vi "MM6.set Special.vi"(0 "i ref in":refnum<vi>, 1 "ms timeout (10000)":i32=10000, 2 "Object":string, 3 "Special":string, 5 "error in (no error)":errorcluster) -> (14 "i ref out":refnum<vi>, 18 "timed out":bool, 19 "error out":errorcluster)   [LabVIEW 2014, in "MM6.lvlib"]
doc: "This VI calls the function \"SetSpecial\" of the object with a certain \"name\" if the Special parameter is not empty nor starting with an asterisk."
uses:
  MM6.lvlib
  CS_Core/CSSystem/CoreDefs/CoreDefs.error_type.ctl
  CS_Core/CSSystem/CoreDefs/CoreDefs.error_severity.ctl
  CS_Core/CSSystem/CoreLib/CoreLib.int 2 byte array.vi
  CS_Core/CSSystem/CoreLib/CoreLib.string 2 byte array.vi
  CS_Core/BaseProcess/BaseProcess.lvlib
  CS_Core/CSSystem/CoreLib/CoreLib.lvlib
  CS_Core/CSSystem/CSSystemLib/CSSystemLib.lvlib
  CSlibraries/UtilityLib/UtilityLib.lvlib
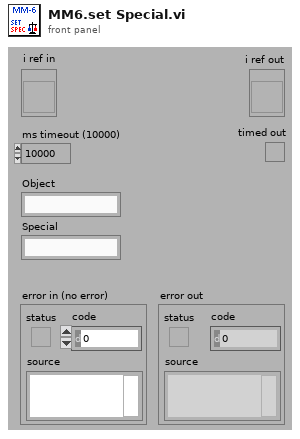
[diagram p1: front panel]
types:
  T1 = typedef "CoreDefs.error_severity.ctl" = enum16{"undefined", "information", "warning", "error", "fatal"}
  T2 = typedef "CoreDefs.error_type.ctl" = enum16{"no error", "can't load process", "can't unload process", "process does not exist", "can't install process", "can't remove process", "unknown function", "time out", "can't execute function", "duplicate queue name", "super not found", "caller queue invalid", "can't ping process", "unknown error", "VISA Error", "VISA timeout", "GPIB timeout", "GPIB error", "communication error", "data type mismatch", "can't read data from OPC server", "can't write data to OPC server", "OET error", "function not implemented", "process already exists", "invalid Shared Variable name", "error writing Shared Variable", "error reading Shared Variable", "invalid client name", "corrupt database", "unknown class", "call not authorized", "parameter out of range", "OET timeout: can't get data to modify", "invalid queue name", "requested operation incompatible with current state", "event undefined", "event disabled", "state undefined", "caller is not a friend", "EventBuilder: bad eventID", "EventBuilder: no DAQ devices", "a thread must not stop itself", "UNUSED ELEMENT4", "DiscArchiver: eventData incomplete", "DiscArchiver: eventData does not belong to run", "DiscArchiver: can't open file", "DiscArchiver: can't write to file", "DiscArchiver: available disc space low", "can't acquire semaphore", "error reading data from database", "notifier object is not existing", "can't register process", "can't unregister process", "illegal event type", "object disabled", "object already exists", "can't change state", "Instrument not found", "no connection to remote node", "invalid reference", "N/A", "UNUSED ELEMENT 1", "element not found", "illegal TCP/IP connection detected", "object does not exist", "invalid access ID", "unknown CS system", "invalid privilige", "unsupported data type", "unsupported server type", "IO server already exists", "Shared Variable already exists"}
  T3 = typedef "CoreDefs.rawDataType.ctl" = i8[]
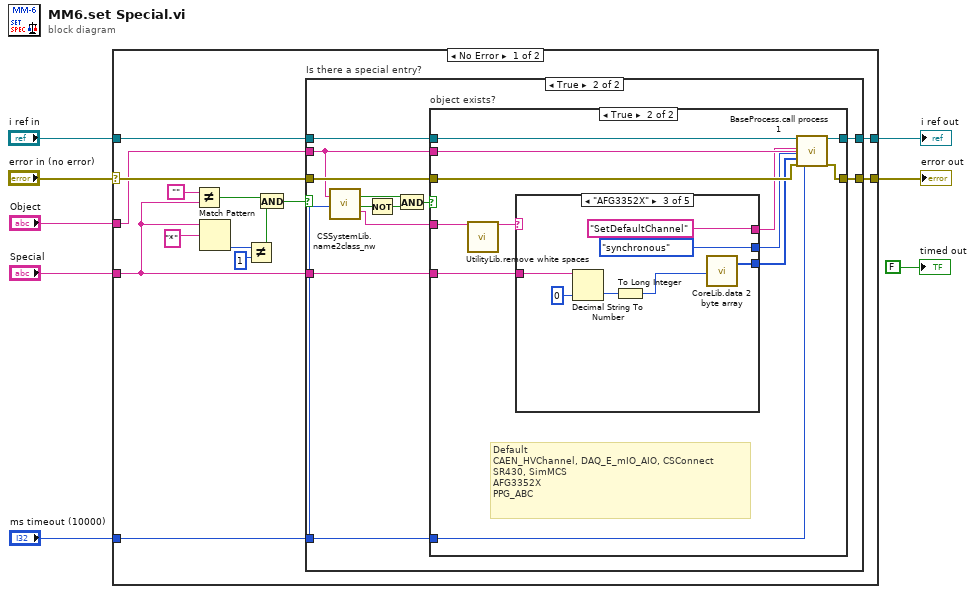
[diagram p0: block diagram]
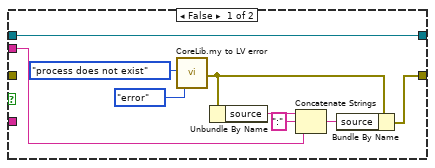
[diagram p3: hidden frame]
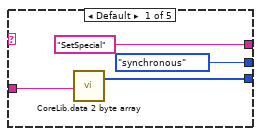
[diagram p4: hidden frame]
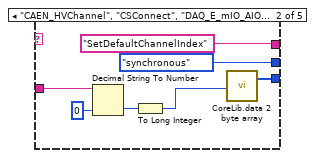
[diagram p5: hidden frame]
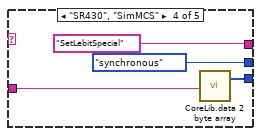
[diagram p6: hidden frame]
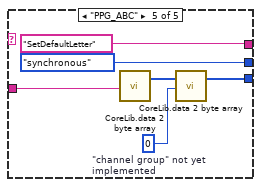
[diagram p7: hidden frame]
diagram:
  n1 = case shown="No Error" "error in (no error)" {
    selector: "error in (no error)" -> [w20 w86]
    tunnel: "i ref in" -> [w21 w87]
    tunnel: [w22 w87] -> w6
    tunnel: [w19 w86] -> w5
    tunnel: "Object" -> [w18 _]
    tunnel: "ms timeout (10000)" -> [w9 _]
    tunnel: "Special" -> [w11 _]
    frame No Error {
      n2 = Not Equal?(x="", y=w11) -> (x != y?=w16:bool)
      n3 = Match Pattern(string=w11, regular expression="*") -> (offset past match=w14:i32)  [unwired: 1 in, 3 out]
      n4 = Not Equal?(x=w14, y=1) -> (x != y?=w17:bool)
      n5 = And(x=w16, y=w17) -> (x .and. y?=w10:bool)
      n6 = case "Is there a special entry?" shown="True" w10 {
        tunnel: [w24 w36] -> w22
        tunnel: w21 -> [w24 w35]
        tunnel: w20 -> [w23 w34]
        tunnel: [w23 w33] -> w19
        tunnel: w18 -> [_ w31]
        tunnel: w11 -> [_ w32]
        tunnel: w9 -> [_ w25]
        frame False {
        }
        frame True {
          n7 = call "CSSystemLib.name2class_nw.vi"("name"=w31, "timeout [ms] (10000)"=w25) -> ("obj exists"=w29:bool, "timed out?"=w30:bool, "classID"=w26:string)  [unwired: 15 in]
          n8 = Not(x=w30) -> (.not. x?=w28:bool)
          n9 = And(x=w29, y=w28) -> (x .and. y?=w27:bool)
          n10 = case "object exists?" shown="True" w27 {
            tunnel: [w45 w57] -> w36
            tunnel: w35 -> [w45 w56]
            tunnel: w34 -> [_ w55]
            tunnel: [w42 w54] -> w33
            tunnel: w32 -> [_ w49]
            tunnel: w31 -> [w38 w53]
            tunnel: w26 -> [_ w48]
            tunnel: w25 -> [_ w46]
            frame False {
              n11 = call "CoreLib.my to LV error.vi"("ErrorTypes"=CoreDefs.error_type."process does not exist", "severityLevel"=CoreDefs.error_severity."error") -> ("myErrorCluster"=w41:errorcluster)  [unwired: 16 in, 1 out]
              n12 = Unbundle By Name(w41) -> ("source"=w40:string)
              n13 = Concatenate Strings(w40, ":" ("string"), w38) -> (w37:string)
              n14 = Bundle By Name(cluster=w41, "source"=w37) -> (w42:errorcluster)
            }
            frame True {
              # "Default\nCAEN_HVChannel, DAQ_E_mIO_AIO, CSConnect\nSR430, SimMCS\nAFG3352X\nPPG_ABC"
              n15 = call "UtilityLib.remove white spaces.vi"("string with blanks"=w48) -> ("string without white spaces"=w47:string)  [unwired: 14 in, 4 out]
              n16 = case shown="\"AFG3352X\"" w47 {
                tunnel: ["SetSpecial" "SetDefaultChannelIndex" "SetDefaultChannel" "SetLebitSpecial" "SetDefaultLetter"] -> w52
                tunnel: [w59 w64 w71 w77 w81] -> w51
                tunnel: [enum16{"simple", "synchronous", "asynchronous"}."synchronous" ("CallType") enum16{"simple", "synchronous", "asynchronous"}."synchronous" ("CallType") enum16{"simple", "synchronous", "asynchronous"}."synchronous" ("CallType") enum16{"simple", "synchronous", "asynchronous"}."synchronous" ("CallType") enum16{"simple", "synchronous", "asynchronous"}."synchronous" ("CallType")] -> w50
                tunnel: w49 -> [w58 w66 w73 w76 w83]
                frame Default {
                  n17 = call-poly "CoreLib.data 2 byte array.vi"("string"=w58) -> ("byteArray out"=w59:T3)  [unwired: 18 in]
                }
                frame "CAEN_HVChannel", "CSConnect", "DAQ_E_mIO_AIO" {
                  n18 = Decimal String To Number(string=w66, default (0L)=0 ("default (0 I32)")) -> (number=w63:i32)  [unwired: 1 in, 1 out]
                  n19 = To Long Integer(number=w63) -> (32bit integer=w62:i32)
                  n20 = call-poly "CoreLib.data 2 byte array.vi"("i32"=w62) -> ("byteArray out"=w64:T3)  [unwired: 18 in]
                }
                frame "AFG3352X" {
                  n21 = Decimal String To Number(string=w73, default (0L)=0 ("default (0 I32)")) -> (number=w70:i32)  [unwired: 1 in, 1 out]
                  n22 = To Long Integer(number=w70) -> (32bit integer=w69:i32)
                  n23 = call-poly "CoreLib.data 2 byte array.vi"("i32"=w69) -> ("byteArray out"=w71:T3)  [unwired: 18 in]
                }
                frame "SR430", "SimMCS" {
                  n24 = call-poly "CoreLib.data 2 byte array.vi"("string"=w76) -> ("byteArray out"=w77:T3)  [unwired: 18 in]
                }
                frame "PPG_ABC" {
                  w80 = 0  # "channel group" not yet implemented
                  n25 = call-poly "CoreLib.data 2 byte array.vi"("string"=w83) -> ("byteArray out"=w82:T3)  [unwired: 18 in]
                  n26 = call-poly "CoreLib.data 2 byte array.vi"("byteArray"=w82, "i32"=w80) -> ("byteArray out"=w81:T3)  [unwired: 17 in]
                }
              }
              n27 = call "BaseProcess.call process 1.vi"("i ref in"=w56, "Object"=w53, "Selector"=w52, "CallType"=w50, "Data"=w51, "error in (no error)"=w55, "timeout (ms)"=w46) -> ("i ref out"=w57:refnum<vi>, "error out"=w54:errorcluster)  [unwired: 10 in, 1 out]
            }
          }
        }
      }
    }
    frame Error {
    }
  }
  "i ref out" <- w6
  "error out" <- w5
  "timed out" <- FALSE ("timed out")
